vi "Custom_Append Front Panel Image to Report (refnum).vi"(0 "report in":refnum<class "NI_report.lvclass">, 1 "alignment (default)":T2, 2 "image format (jpeg)":enum32{"PNG", "JPEG", "GIF"}(ring)=enum."JPEG", 5 "VI":refnum<vi>, 9 "description":string, 11 "error in (no error)":errorcluster, 12 "visible area only?":bool, 13 "MS Office parameters":T1) -> (4 "report out":refnum<class "NI_report.lvclass">, 6 "VI out":refnum<vi>, 8 "start out (Word)":i32, 10 "end out (Word)":i32, 15 "error out":errorcluster)   [LabVIEW 2019]
doc: "Creates an image of the front panel of the VI you specify in <B>VI</B> and appends it to a report. Wire data to the <B>VI</B> input to determine the polymorphic instance to use or manually select the instance."
uses:
  <vilib>/Utility/NIReport.llb/NI_report.lvclass
  <vilib>/Utility/NIReport.llb/HTML Report Image Alignment.ctl
  <vilib>/Utility/NIReport.llb/NI_ReportGenerationCore.lvlib
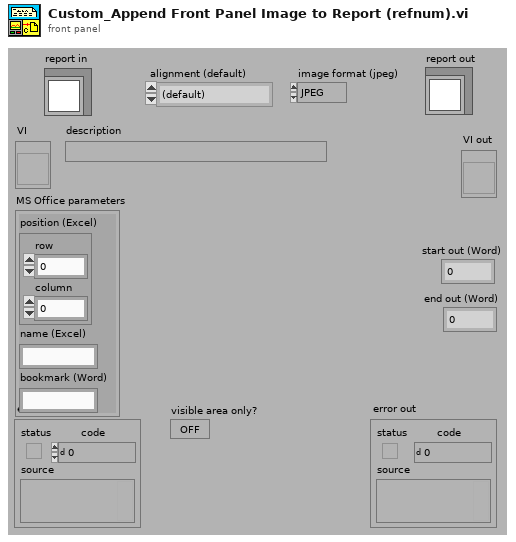
[diagram p1: front panel]
types:
  T1 = cluster{"position (Excel)":cluster{"row":i32, "column":i32}, "name (Excel)":string, "bookmark (Word)":string}
  T2 = typedef "NI_ReportGenerationCore.lvlib/HTML Report Image Alignment.ctl" = enum16{"(default)", "LEFT", "RIGHT", "TOP", "TEXTTOP", "MIDDLE", "ABSMIDDLE", "BASELINE", "BOTTOM", "ABSBOTTOM"}
  T3 = typedef "imagedata.ctl" = cluster{"image type":i32, "image depth":i32, "image":u8[], "mask":u8[], "colors":u32[], "Rectangle":cluster{"left":i16, "top":i16, "right":i16, "bottom":i16}}
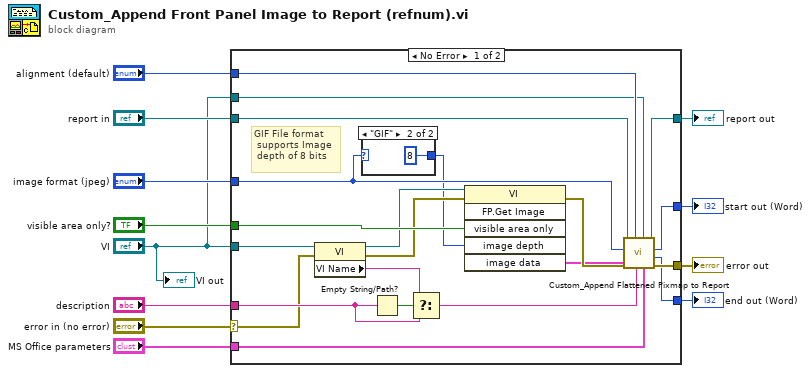
[diagram p0: block diagram]
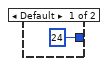
[diagram p2: hidden frame]
diagram:
  n1 = case shown="No Error" "error in (no error)" {
    selector: "error in (no error)" -> [w23 w37]
    tunnel: "description" -> [w33 _]
    tunnel: "visible area only?" -> [w32 _]
    tunnel: "VI" -> [w31 _]
    tunnel: "image format (jpeg)" -> [w19 _]
    tunnel: [w24 w37] -> w6
    tunnel: [w15 w36] -> w7
    tunnel: "alignment (default)" -> [w26 _]
    tunnel: "report in" -> [w14 w36]
    tunnel: "MS Office parameters" -> [w21 _]
    tunnel: [w17 _] -> w3
    tunnel: [w16 _] -> w2
    tunnel: "VI" -> [w13 _]
    frame No Error {
      # "GIF File format\n supports Image\n depth of 8 bits"
      n2 = property class="VI"(reference=w31, error in=w23) -> (reference out=w28:refnum<vi>, error out=w27:errorcluster, "VI Name"=w29:string)
      n3 = case shown="\"GIF\"" w19 {
        tunnel: [24 ("image depth") 8 ("image depth")] -> w18
        frame Default {
        }
        frame "GIF" {
        }
      }
      n4 = Empty String/Path?(string/path=w33) -> (empty?=w30:bool)
      n5 = Select(t=w29, s=w30, f=w33) -> (s? t:f=w22:string)
      n6 = invoke class="VI" method="FP.Get Image"(reference=w28, error in=w27, "visible area only"=w32, "image depth"=w18) -> (error out=w25:errorcluster, "image data"=w20:T3)  [unwired: 2 in, 4 out]
      n7 = call "Custom_Append Flattened Pixmap to Report.vi"("MS Office parameters"=w21, "VI"=w13, "caption or alt string"=w22, "alignment (default)"=w26, "error in (no error)"=w25, "image data"=w20, "image format (jpeg)"=w19, "report in"=w14) -> ("error out"=w24:errorcluster, "end out (word)"=w16:i32, "start out (word)"=w17:i32, "report out"=w15:refnum<class "NI_report.lvclass">)
    }
    frame Error {
    }
  }
  "error out" <- w6
  "report out" <- w7
  "start out (Word)" <- w3
  "end out (Word)" <- w2
  "VI out" <- "VI"
